vi "SaveVolt (SubVI).vi"(11 "Protocol":refnum<vi>) -> ()   [LabVIEW 2017]
uses:
  <vilib>/Utility/file.llb/Write Delimited Spreadsheet (string).vi
panel:
  out "error out":errorcluster
  in  "delimiter (\\t)":string="\t"
  in  "Discription":string[](array[string])=["Время", "Uскз А, В", "Uскз B, В", "Fа, кГц", "Fb, кГц", "Диап. A", "Диап. B", "Прим."]
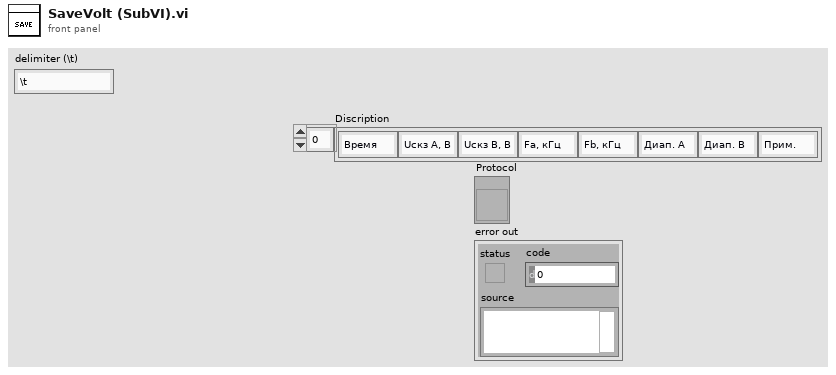
[diagram p1: front panel]
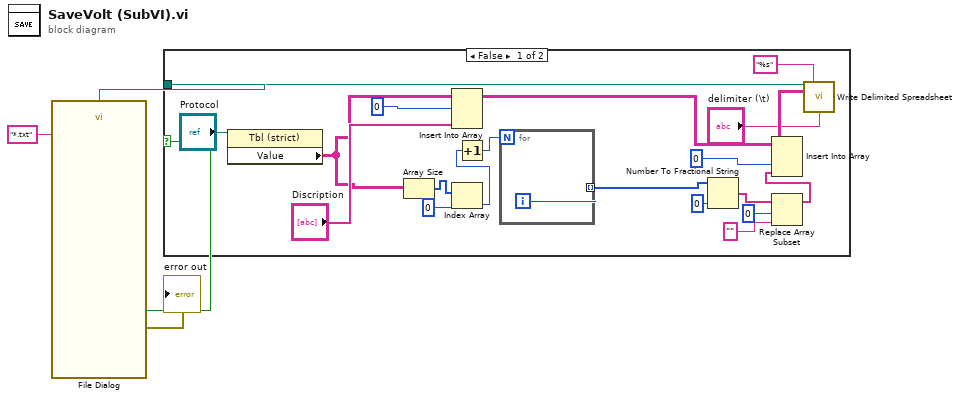
[diagram p0: block diagram]
diagram:
  n1 = call "File Dialog"("pattern (all files)"="*.txt") -> ("selected path"=w4:path, "cancelled"=w3:bool, "error out"=→"error out":errorcluster)  [unwired: 11 in, 1 out]
  n2 = case shown="False" w3 {
    tunnel: w4 -> [w24 _]
    frame False {
      n3 = property class="Tbl (strict)"(reference="Protocol") -> ("Value"=w7:string[][])  [unwired: 1 in, 2 out]
      n4 = Array Size(array=w7) -> (size(s)=w21:i32[])
      n5 = Insert Into Array(array=w7, index (row)=0, new element="Discription") -> (w19:string[][])  [unwired: 1 in]
      n6 = Index Array(array=w21, index=0) -> (element=w6:i32)
      n7 = Increment(x=w6) -> (x+1=w5:i32)
      n8 = for {
        N: w5 -> [_]
        tunnel: [w25] -> w16 mode=indexing
        i -> [w25]
      }
      n9 = Number To Fractional String(number=w16, precision (6)=i16 0) -> (F-format string=w14:string[])  [unwired: 2 in]
      n10 = Replace Array Subset(array=w14, new element="" ("new element/subarray"), index=0) -> (w13:string[])
      n11 = Insert Into Array(array=w19, index (col)=0 ("disabled index (col)"), new element=w13) -> (w17:string[][])  [unwired: 1 in]
      n12 = call-poly <vilib>:"Write Delimited Spreadsheet.vi"("file path (dialog if empty)"=w24, "format (%s)"="%s", "2D data"=w17, "delimiter (\\t)"="delimiter (\\t)") -> ()  [unwired: 10 in, 2 out]
    }
    frame True {
    }
  }
